vi "CLD 11 Producer consumer events front panel.vi"() -> ()   [LabVIEW 2018]
doc: "CLD 11 exercise"
uses:
  CLD 11 Producer Consumer Data Structure.ctl
  CLD 11 CSV file data structure.ctl
  CLD 11 producer consumer enum.ctl
  CLD 11 CSV file enum.ctl
panel:
  out "Current Time target":dbl
  out "Step 3":bool
  out "Step 2":bool
  out "Step 1":bool
  out "Time Has Elapsed":bool
  out "Elapsed Time":string
  in  "Auto Reset":bool=TRUE
  in  "Reset Button":bool
  in  "Stop VI":bool
  in  "Time Target (s)":dbl
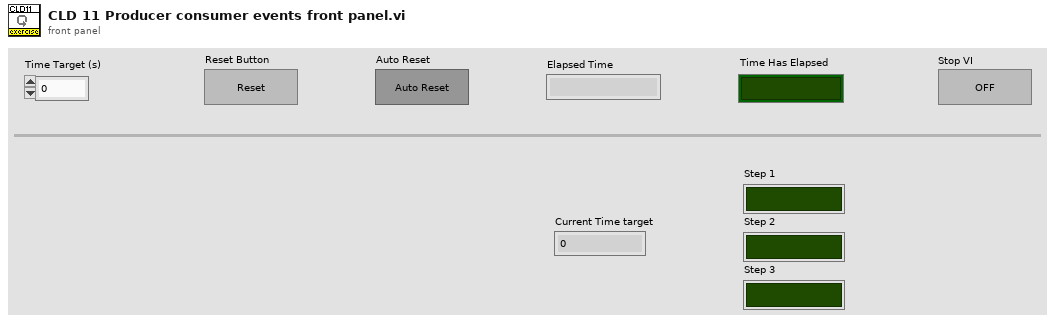
[diagram p1: front panel]
types:
  T1 = typedef "CLD 11 CSV file data structure.ctl" = cluster{"Dwell Time":i32, "State 1":bool, "State 2":bool, "State 3":bool}
  T2 = typedef "CLD 11 producer consumer enum.ctl" = enum16{"Initialize App", "Read CSV File", "Check Timer", "Run State One", "Run State Two", "Run State Three", "Stop App", "Reset", "Autoreset"}
  T3 = typedef "CLD 11 Producer Consumer Data Structure.ctl" = cluster{"CSV File Data Structure":T1, "Time has Elapsed":bool, "Reset":bool, "Autoreset":bool, "Time Target (s)":dbl, "Current State Number":i32}
  T4 = typedef "CLD 11 CSV file enum.ctl" = enum16{"Read CSV", "Write CSV"}
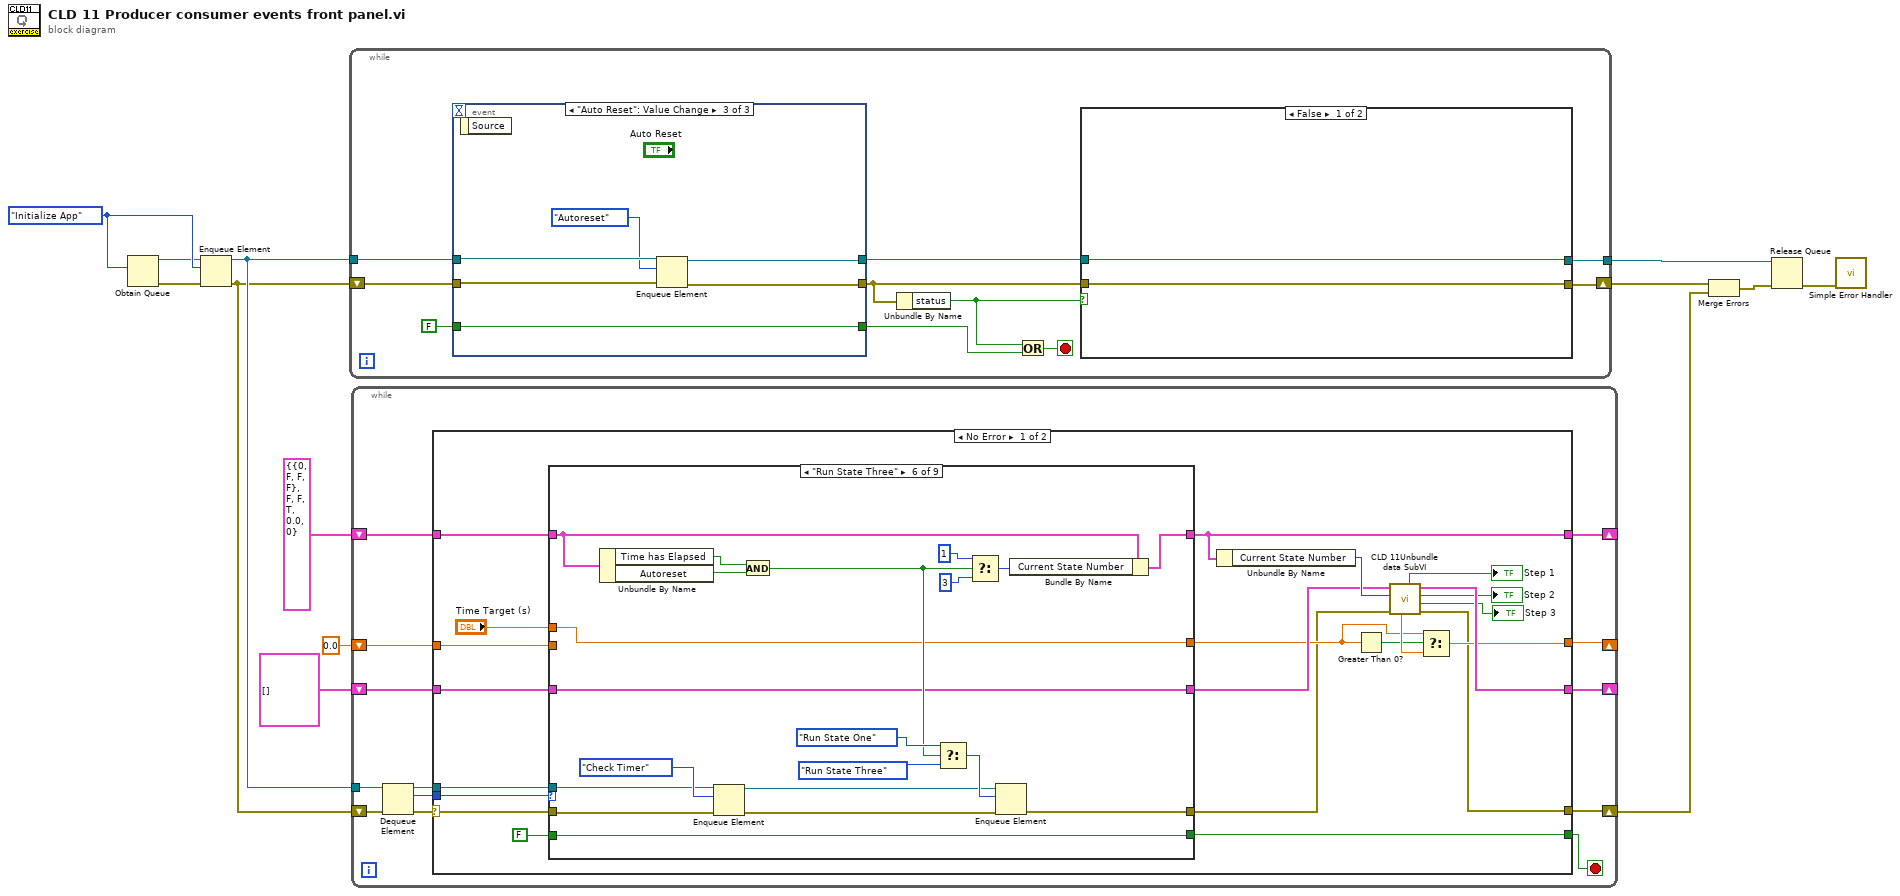
[diagram p0: block diagram]
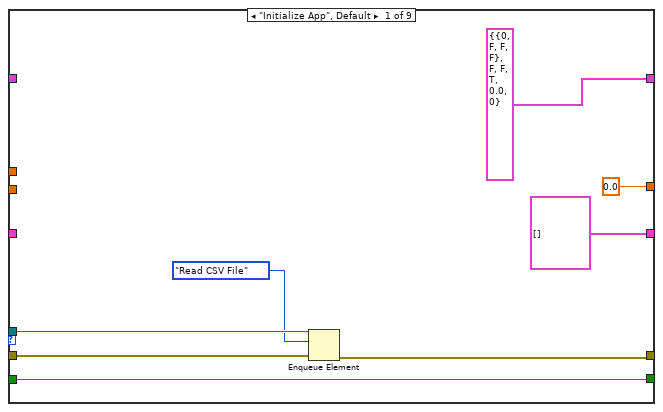
[diagram p2: hidden frame]
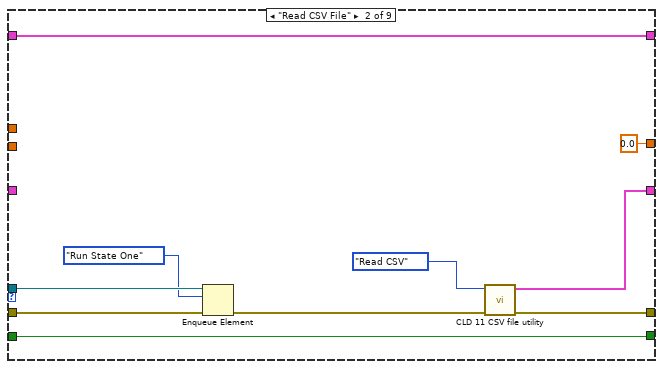
[diagram p3: hidden frame]
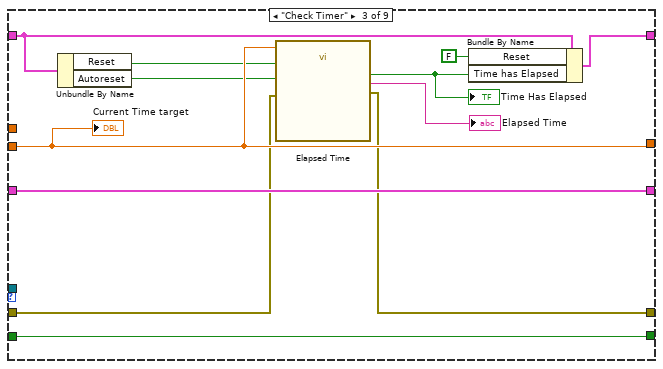
[diagram p4: hidden frame]
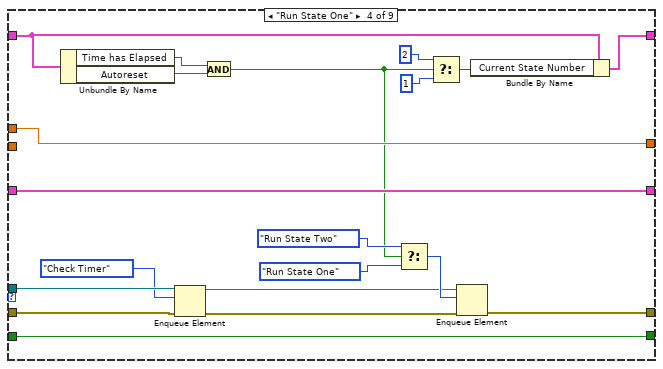
[diagram p5: hidden frame]
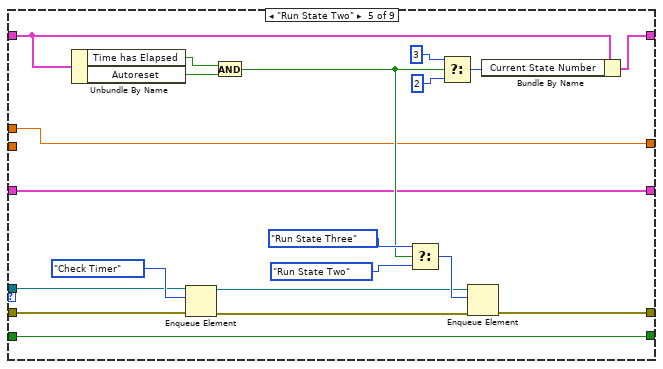
[diagram p6: hidden frame]
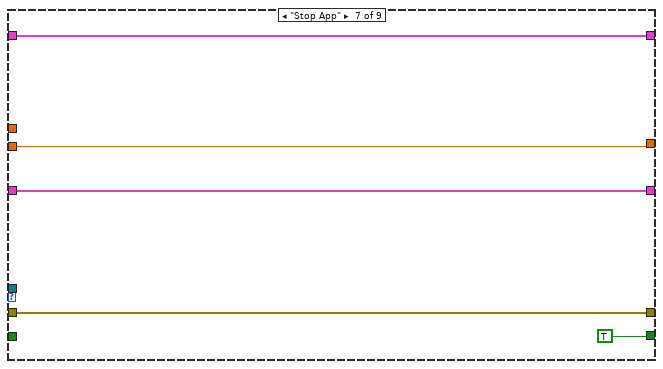
[diagram p7: hidden frame]
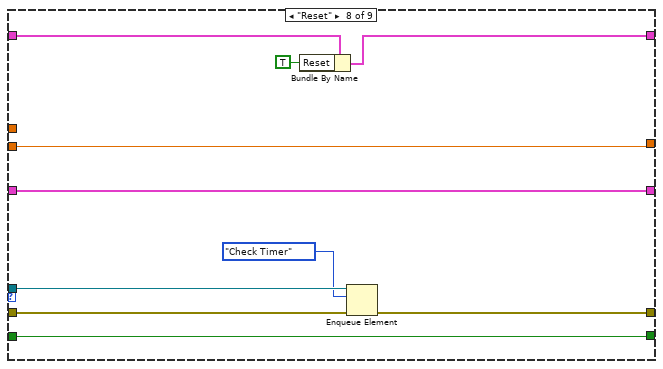
[diagram p8: hidden frame]
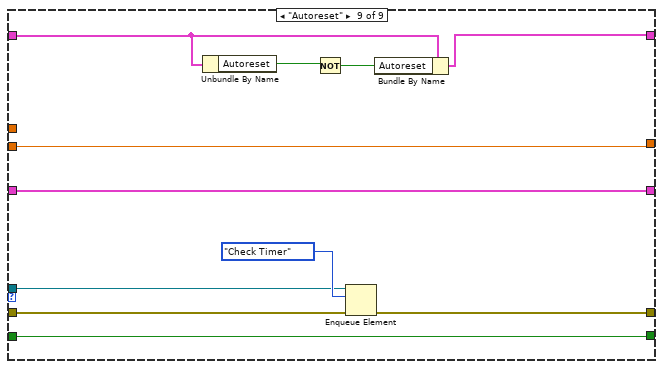
[diagram p9: hidden frame]
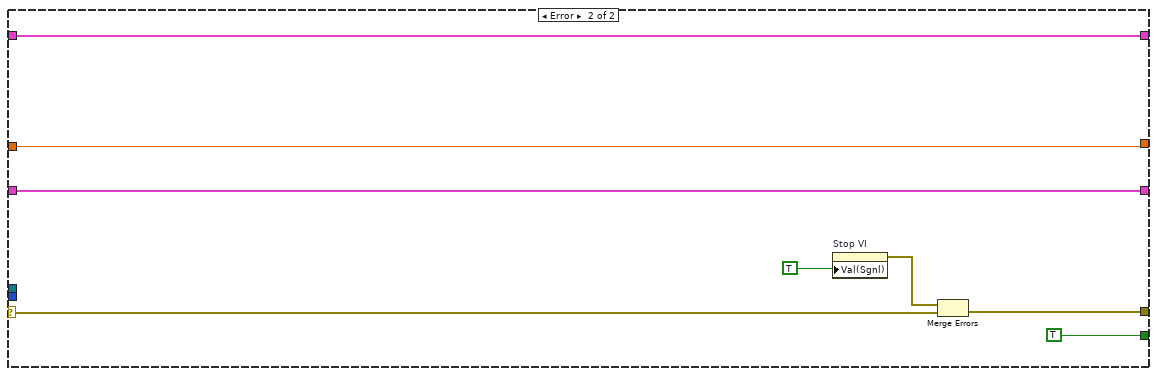
[diagram p10: hidden frame]
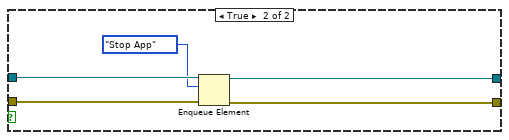
[diagram p11: hidden frame]
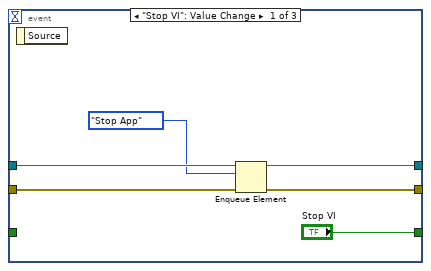
[diagram p12: hidden frame]
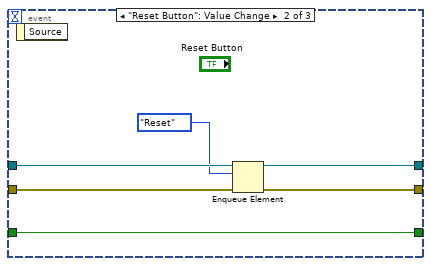
[diagram p13: hidden frame]
diagram:
  w13 = CLD_11_producer_consumer_enum."Initialize App" ("CLD 11 Timer Enum")
  n1 = Obtain Queue(element data type=w13) -> (queue out=w12:refnum<queue>, error out=w10:errorcluster)  [unwired: 4 in, 1 out]
  n2 = Enqueue Element(queue=w12, element=w13, error in (no error)=w10) -> (queue out=w11:refnum<queue>, error out=w5:errorcluster)  [unwired: 1 in, 1 out]
  n3 = while {
    tunnel: w11 -> [w22]
    shift-right: [w15] -> w9
    shift-left: w5 -> [w23]
    tunnel: [w14] -> w7
    stop <- w20 stop-if-true
    n4 = event shown="[2] \"Auto Reset\": Value Change" {
      selector: _ -> [_ _ _]
      dyn-events: _ -> [_ _ _]
      timeout: _ -> [_ _ _]
      tunnel: ["Stop VI" w42 w43] -> w18
      tunnel: w23 -> [w35 w41 w48]
      tunnel: w22 -> [w34 w39 w46]
      tunnel: [w32 w40 w47] -> w16
      tunnel: [w31 w38 w45] -> w21
      tunnel: FALSE -> [_ w42 w43]
      event "Stop VI": Value Change {
        n5 = event-data() -> ()  [unwired: 1 in, 1 out]
        n6 = Enqueue Element(queue=w34, element=CLD_11_producer_consumer_enum."Stop App" ("CLD 11 Timer Enum"), error in (no error)=w35) -> (queue out=w31:refnum<queue>, error out=w32:errorcluster)  [unwired: 1 in, 1 out]
      }
      event "Reset Button": Value Change {
        n7 = event-data() -> ()  [unwired: 1 in, 1 out]
        n8 = Enqueue Element(queue=w39, element=CLD_11_producer_consumer_enum."Reset", error in (no error)=w41) -> (queue out=w38:refnum<queue>, error out=w40:errorcluster)  [unwired: 1 in, 1 out]
      }
      event "Auto Reset": Value Change {
        n9 = event-data() -> ()  [unwired: 1 in, 1 out]
        n10 = Enqueue Element(queue=w46, element=CLD_11_producer_consumer_enum."Autoreset", error in (no error)=w48) -> (queue out=w45:refnum<queue>, error out=w47:errorcluster)  [unwired: 1 in, 1 out]
      }
    }
    n11 = Unbundle By Name(w16) -> ("status"=w19:bool)
    n12 = Or(x=w19, y=w18) -> (x .or. y?=w20:bool)
    n13 = case shown="False" w19 {
      tunnel: w21 -> [w25 w28]
      tunnel: w16 -> [w24 w30]
      tunnel: [w24 w29] -> w15
      tunnel: [w25 w27] -> w14
      frame False {
      }
      frame True {
        n14 = Enqueue Element(queue=w28, element=CLD_11_producer_consumer_enum."Stop App", error in (no error)=w30) -> (queue out=w27:refnum<queue>, error out=w29:errorcluster)  [unwired: 1 in, 1 out]
      }
    }
  }
  n15 = while {
    tunnel: w11 -> [w61]
    shift-right: [w58] -> w4
    shift-left: w5 -> [w60]
    shift-right: [w51] -> _
    shift-left: T3 {"CSV File Data Structure"={"Dwell Time"=0, "State 1"=FALSE, "State 2"=FALSE, "State 3"=FALSE}, "Time has Elapsed"=FALSE, "Reset"=FALSE, "Autoreset"=TRUE, "Time Target (s)"=0.0, "Current State Number"=0} ("Producer Consumer Data Structure") -> [w52]
    shift-right: [w50] -> _
    shift-left: 0.0 -> [w53]
    shift-right: [w49] -> _
    shift-left: T1[] [] -> [w54]
    stop <- w57 stop-if-true
    n16 = Dequeue Element(queue=w61, error in (no error)=w60) -> (queue out=w55:refnum<queue>, element=w56:T2, error out=w59:errorcluster)  [unwired: 1 in, 1 out]
    n17 = case shown="No Error" w59 {
      selector: w59 -> [w81 w206]
      tunnel: [w64 w204] -> w58
      tunnel: [w63 TRUE] -> w57
      tunnel: w56 -> [w83 _]
      tunnel: w55 -> [w82 _]
      tunnel: w54 -> [w80 w200]
      tunnel: w53 -> [w79 w201]
      tunnel: w52 -> [w77 w202]
      tunnel: [w76 w202] -> w51
      tunnel: [w69 w201] -> w50
      tunnel: [w73 w200] -> w49
      frame No Error {
        n18 = case shown="\"Run State Three\"" w83 {
          tunnel: w82 -> [w85 w93 _ w120 w139 w159 _ w181 w192]
          tunnel: w81 -> [w87 w95 w104 w122 w138 w158 w177 w183 w191]
          tunnel: w80 -> [_ _ w113 w117 w136 w156 w176 w184 w193]
          tunnel: w79 -> [_ _ w112 _ _ _ w175 w188 w194]
          tunnel: "Time Target (s)" -> [_ _ _ w116 w135 w155 _ _ _]
          tunnel: w77 -> [_ w100 w109 w133 w142 w163 w174 w187 w196]
          tunnel: [T1[] [] w98 w113 w117 w136 w156 w176 w184 w193] -> w74
          tunnel: [T3 {"CSV File Data Structure"={"Dwell Time"=0, "State 1"=FALSE, "State 2"=FALSE, "State 3"=FALSE}, "Time has Elapsed"=FALSE, "Reset"=FALSE, "Autoreset"=TRUE, "Time Target (s)"=0.0, "Current State Number"=0} ("Producer Consumer Data Structure") w100 w108 w132 w143 w162 w174 w186 w195] -> w76
          tunnel: [0.0 0.0 w112 w116 w135 w155 w175 w188 w194] -> w70
          tunnel: [w86 w97 w103 w126 w137 w157 w177 w182 w190] -> w65
          tunnel: [w88 w96 w102 w114 w134 w154 TRUE w179 w189] -> w63
          tunnel: FALSE -> [w88 w96 w102 w114 w134 w154 _ w179 w189]
          frame "Initialize App", Default {
            n19 = Enqueue Element(queue=w85, element=CLD_11_producer_consumer_enum."Read CSV File", error in (no error)=w87) -> (error out=w86:errorcluster)  [unwired: 1 in, 2 out]
          }
          frame "Read CSV File" {
            n20 = Enqueue Element(queue=w93, element=CLD_11_producer_consumer_enum."Run State One", error in (no error)=w95) -> (error out=w94:errorcluster)  [unwired: 1 in, 2 out]
            n21 = call "CLD 11 CSV file utility.vi"("Error In"=w94, "CSV File Enum"=CLD_11_CSV_file_enum."Read CSV") -> ("Error Out"=w97:errorcluster, "[Data Out]"=w98:T1[])  [unwired: 8 in]
          }
          frame "Check Timer" {
            n22 = Unbundle By Name(w109) -> ("Reset"=w111:bool, "Autoreset"=w110:bool)
            n23 = call "Elapsed Time"("Time Target (s)"=w112, "Reset"=w111, "Auto Reset"=w110, "error in (no error)"=w104) -> ("Time has Elapsed"=w106:bool, "Elapsed Time Text"=→"Elapsed Time":string, "error out"=w103:errorcluster)  [unwired: 8 in, 5 out]
            "Time Has Elapsed" <- w106
            n24 = Bundle By Name(cluster=w109, "Reset"=FALSE, "Time has Elapsed"=w106) -> (w108:T3)
            "Current Time target" <- w112
          }
          frame "Run State One" {
            n25 = Unbundle By Name(w133) -> ("Time has Elapsed"=w131:bool, "Autoreset"=w130:bool)
            n26 = Enqueue Element(queue=w120, element=CLD_11_producer_consumer_enum."Check Timer" ("CLD 11 Timer Enum"), error in (no error)=w122) -> (queue out=w119:refnum<queue>, error out=w121:errorcluster)  [unwired: 1 in, 1 out]
            n27 = And(x=w131, y=w130) -> (x .and. y?=w115:bool)
            n28 = Select(t=CLD_11_producer_consumer_enum."Run State Two" ("CLD 11 Timer Enum"), s=w115, f=CLD_11_producer_consumer_enum."Run State One" ("CLD 11 Timer Enum")) -> (s? t:f=w125:T2)
            n29 = Select(t=2, s=w115, f=1) -> (s? t:f=w129:i32)
            n30 = Enqueue Element(queue=w119, element=w125, error in (no error)=w121) -> (error out=w126:errorcluster)  [unwired: 1 in, 2 out]
            n31 = Bundle By Name(cluster=w133, "Current State Number"=w129) -> (w132:T3)
          }
          frame "Run State Two" {
            n32 = Unbundle By Name(w142) -> ("Time has Elapsed"=w141:bool, "Autoreset"=w140:bool)
            n33 = Enqueue Element(queue=w139, element=CLD_11_producer_consumer_enum."Check Timer" ("CLD 11 Timer Enum"), error in (no error)=w138) -> (queue out=w146:refnum<queue>, error out=w147:errorcluster)  [unwired: 1 in, 1 out]
            n34 = And(x=w141, y=w140) -> (x .and. y?=w144:bool)
            n35 = Select(t=CLD_11_producer_consumer_enum."Run State Three" ("CLD 11 Timer Enum"), s=w144, f=CLD_11_producer_consumer_enum."Run State Two" ("CLD 11 Timer Enum")) -> (s? t:f=w150:T2)
            n36 = Select(t=3, s=w144, f=2) -> (s? t:f=w153:i32)
            n37 = Enqueue Element(queue=w146, element=w150, error in (no error)=w147) -> (error out=w137:errorcluster)  [unwired: 1 in, 2 out]
            n38 = Bundle By Name(cluster=w142, "Current State Number"=w153) -> (w143:T3)
          }
          frame "Run State Three" {
            n39 = Unbundle By Name(w163) -> ("Time has Elapsed"=w161:bool, "Autoreset"=w160:bool)
            n40 = Enqueue Element(queue=w159, element=CLD_11_producer_consumer_enum."Check Timer" ("CLD 11 Timer Enum"), error in (no error)=w158) -> (queue out=w166:refnum<queue>, error out=w167:errorcluster)  [unwired: 1 in, 1 out]
            n41 = And(x=w161, y=w160) -> (x .and. y?=w164:bool)
            n42 = Select(t=CLD_11_producer_consumer_enum."Run State One" ("CLD 11 Timer Enum"), s=w164, f=CLD_11_producer_consumer_enum."Run State Three" ("CLD 11 Timer Enum")) -> (s? t:f=w170:T2)
            n43 = Select(t=1, s=w164, f=3) -> (s? t:f=w173:i32)
            n44 = Enqueue Element(queue=w166, element=w170, error in (no error)=w167) -> (error out=w157:errorcluster)  [unwired: 1 in, 2 out]
            n45 = Bundle By Name(cluster=w163, "Current State Number"=w173) -> (w162:T3)
          }
          frame "Stop App" {
          }
          frame "Reset" {
            n46 = Bundle By Name(cluster=w187, "Reset"=TRUE) -> (w186:T3)
            n47 = Enqueue Element(queue=w181, element=CLD_11_producer_consumer_enum."Check Timer", error in (no error)=w183) -> (error out=w182:errorcluster)  [unwired: 1 in, 2 out]
          }
          frame "Autoreset" {
            n48 = Unbundle By Name(w196) -> ("Autoreset"=w198:bool)
            n49 = Not(x=w198) -> (.not. x?=w197:bool)
            n50 = Enqueue Element(queue=w192, element=CLD_11_producer_consumer_enum."Check Timer", error in (no error)=w191) -> (error out=w190:errorcluster)  [unwired: 1 in, 2 out]
            n51 = Bundle By Name(cluster=w196, "Autoreset"=w197) -> (w195:T3)
          }
        }
        n52 = Unbundle By Name(w76) -> ("Current State Number"=w75:i32)
        n53 = Greater Than 0?(x=w70) -> (x > 0?=w71:bool)
        n54 = call "CLD 11Unbundle data SubVI.vi"("error in (no error)"=w65, "Current State Number"=w75, "[Data In]"=w74) -> ("error out"=w64:errorcluster, "State 3"=→"Step 3":bool, "State 2"=→"Step 2":bool, "[Data Out]"=w73:T1[], "State 1"=→"Step 1":bool, "Dwell Time"=w72:dbl)  [unwired: 2 in, 1 out]
        n55 = Select(t=w70, s=w71, f=w72) -> (s? t:f=w69:dbl)
      }
      frame Error {
        n56 = property on="Stop VI" class="Bool"("Val(Sgnl)"=TRUE) -> (error out=w205:errorcluster)  [unwired: 2 in, 1 out]
        n57 = Merge Errors(w205, w206) -> (w204:errorcluster)
      }
    }
  }
  n58 = Merge Errors(w9, w4) -> (w8:errorcluster)
  n59 = Release Queue(queue=w7, error in (no error)=w8) -> (error out=w6:errorcluster)  [unwired: 1 in, 2 out]
  n60 = call <vilib>:"Simple Error Handler.vi"("error in (no error)"=w6) -> ()  [unwired: 4 in, 5 out]
